vi "Create_file_diag.vi"(8 "error in (no error)":errorcluster, 11 "Comment":string) -> (0 "error out":errorcluster, 3 "Measurement File out":path)   [LabVIEW 2015]
uses:
  Global 1_diag.vi
  <vilib>/Utility/file.llb/Write To Spreadsheet File (string).vi
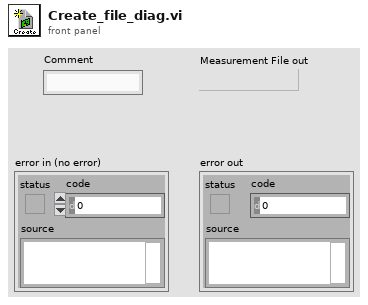
[diagram p1: front panel]
types:
  T1 = enum16{"open", "replace", "create", "open or create", "replace or create", "replace or create with confirmation"}
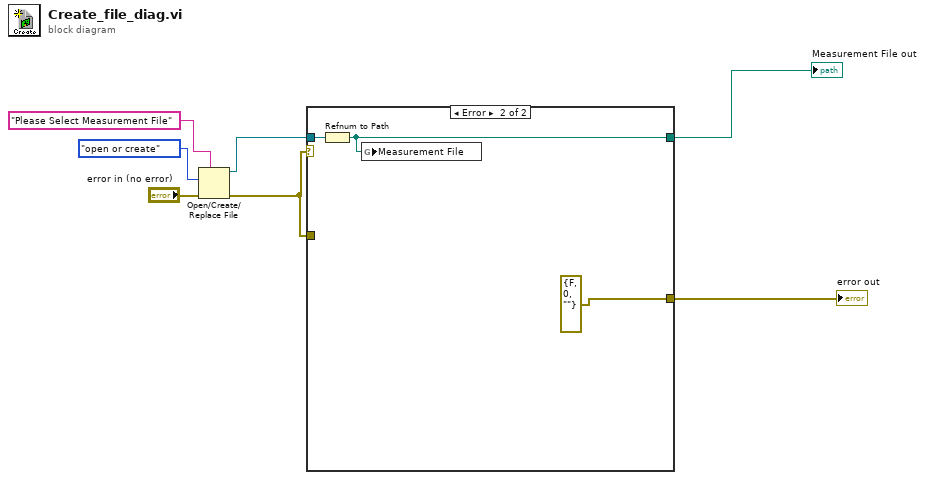
[diagram p0: block diagram]
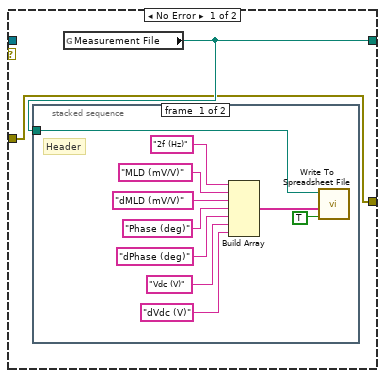
[diagram p2: hidden frame]
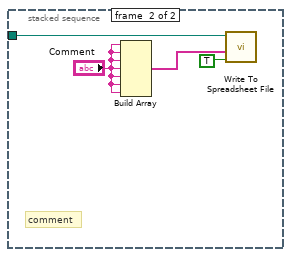
[diagram p3: hidden frame]
diagram:
  n1 = Open/Create/Replace File(error in="error in (no error)", prompt="Please Select Measurement File", operation (0:open)=T1."open or create") -> (refnum out=w5:refnum<file>, error out=w2:errorcluster)  [unwired: 3 in, 1 out]
  n2 = case shown="Error" w2 {
    tunnel: w5 -> [_ w26]
    tunnel: [w9 w25] -> w3
    tunnel: w2 -> [w8 _]
    tunnel: [w8 errorcluster {"status"=FALSE, "code"=0, "source"=""} ("error constant")] -> w1
    frame No Error {
      n3 = global read "Global 1_diag.vi" "Measurement File"() -> (w9:path)
      n4 = stacked-sequence {
        tunnel: w9 -> [w10 w20]
        frame #0 {
          # "Header"
          n5 = Build Array("2f (Hz)", "MLD (mV/V)", "dMLD (mV/V)", "Phase (deg)", "dPhase (deg)", "Vdc (V)", "dVdc (V)") -> (w12:string[])
          n6 = call-poly <vilib>:"Write To Spreadsheet File.vi"("append to file? (new file:F)"=TRUE, "1D data"=w12, "file path (dialog if empty)"=w10) -> ()  [unwired: 5 in, 1 out]
        }
        frame #1 {
          # "comment"
          n7 = Build Array("Comment", "Comment", "Comment", "Comment", "Comment", "Comment", "Comment") -> (w23:string[])
          n8 = call-poly <vilib>:"Write To Spreadsheet File.vi"("append to file? (new file:F)"=TRUE, "1D data"=w23, "file path (dialog if empty)"=w20) -> ()  [unwired: 5 in, 1 out]
        }
      }
    }
    frame Error {
      n9 = Refnum to Path(1:w26) -> (0:w25:path)
      n10 = global write "Global 1_diag.vi" "Measurement File"(w25) -> ()
    }
  }
  "Measurement File out" <- w3
  "error out" <- w1
